vi "读取数据文件-扭转.vi"(0 "文件路径（使用对话框）":path) -> (1 "第一列":dbl[](array[numeric]), 2 "第二列":dbl[](array[numeric]))   [LabVIEW 2016]
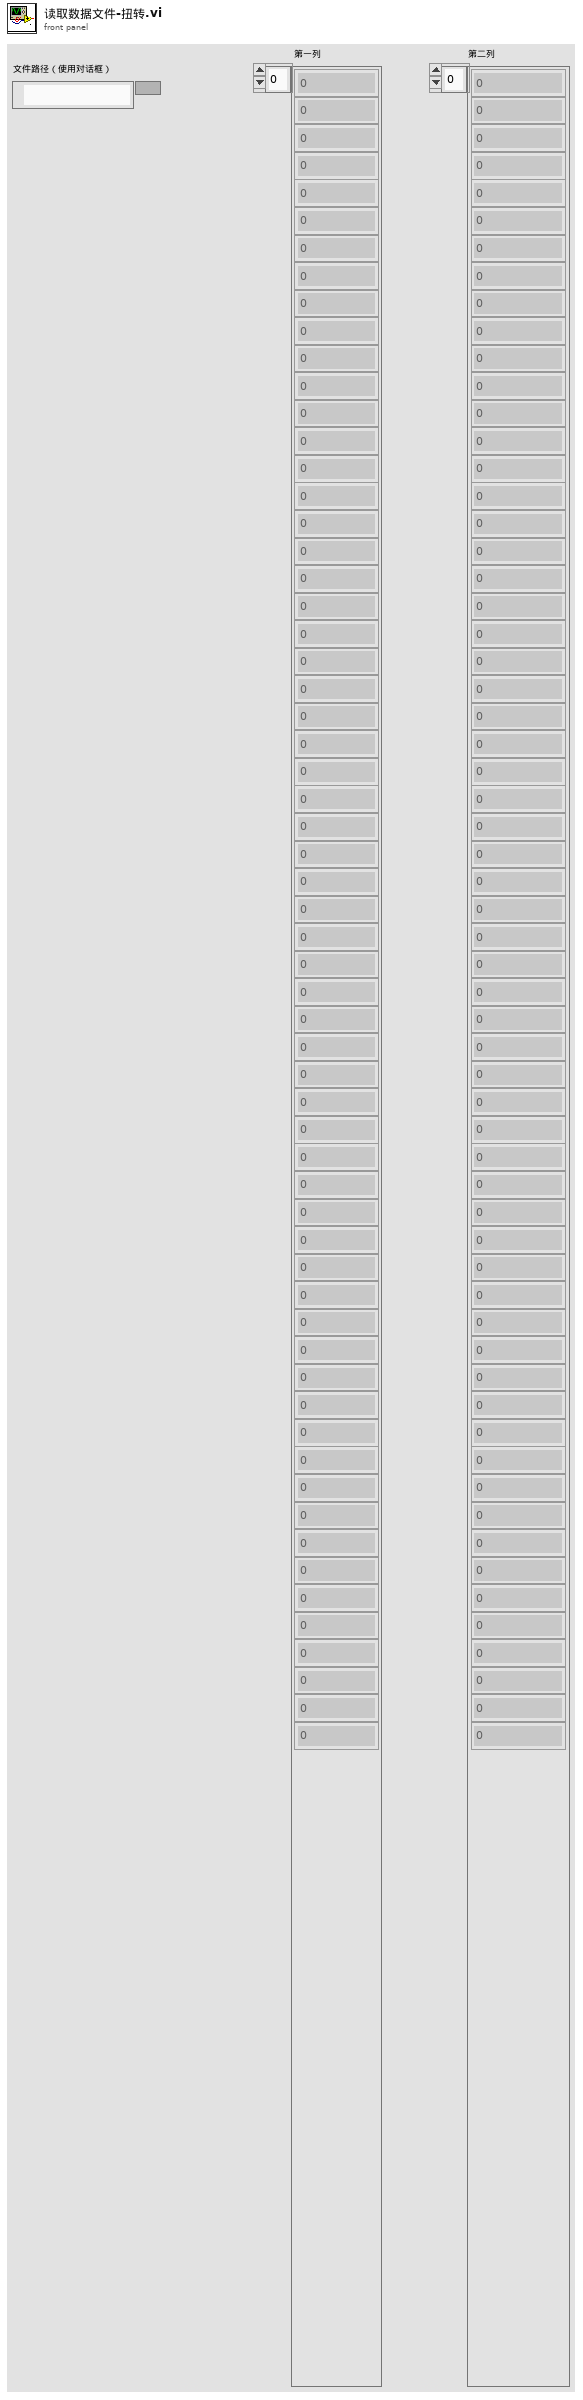
[diagram p1: front panel]
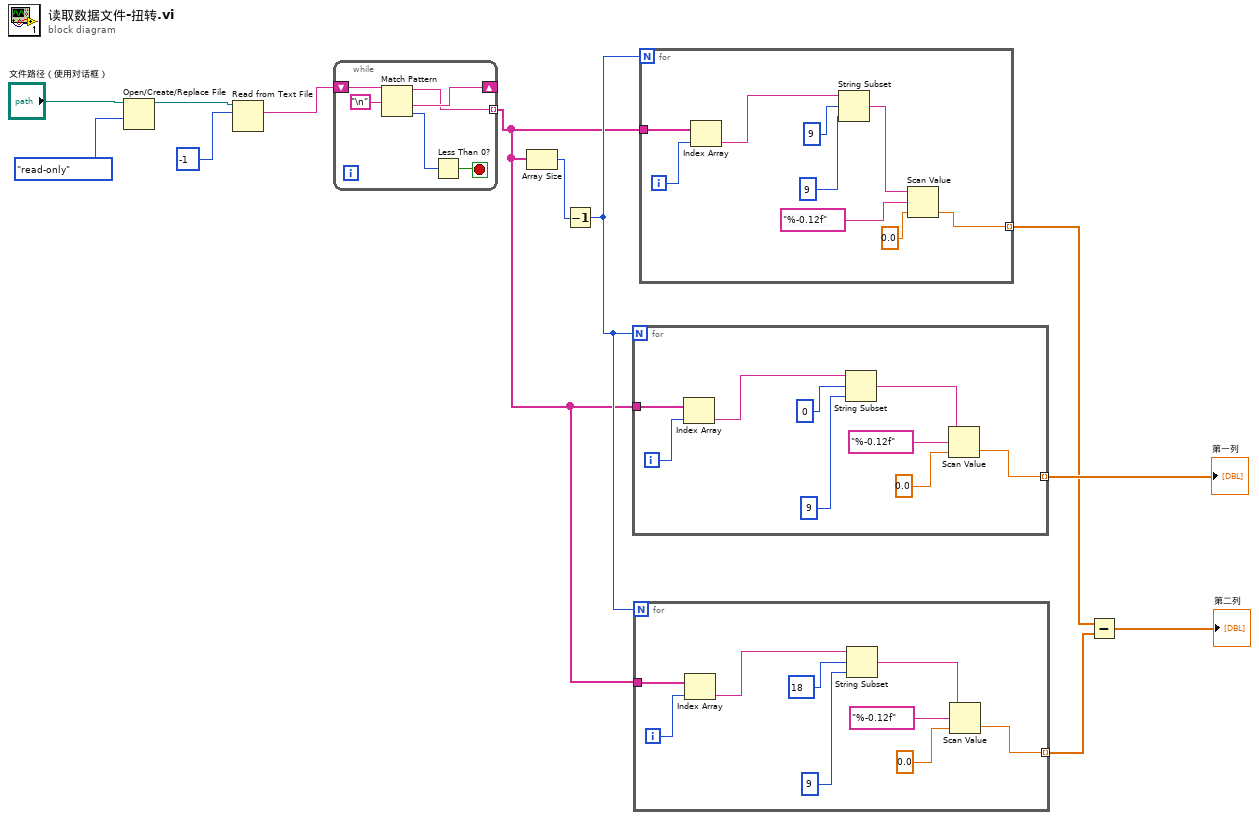
[diagram p0: block diagram]
diagram:
  n1 = Open/Create/Replace File(file path (use dialog)="文件路径（使用对话框）", access (0:read/write)=enum16{"read/write", "read-only", "write-only"}."read-only" ("权限(0:read/write)")) -> (refnum out=w10:refnum<file>)  [unwired: 4 in, 2 out]
  n2 = Read from Text File(file (use dialog)=w10, count=-1 ("计数")) -> (text=w8:string)  [unwired: 2 in, 3 out]
  n3 = while {
    tunnel: [w13] -> w4 mode=indexing
    shift-right: [w16] -> _
    shift-left: w8 -> [w17]
    stop <- w15 stop-if-true
    n4 = Match Pattern(string=w17, regular expression="\n") -> (before substring=w13:string, after substring=w16:string, offset past match=w14:i32)  [unwired: 1 in, 1 out]
    n5 = Less Than 0?(x=w14) -> (x < 0?=w15:bool)
  }
  n6 = Array Size(array=w4) -> (size(s)=w7:i32)
  n7 = Decrement(x=w7) -> (x-1=w5:i32)
  n8 = for {
    N: w5 -> [_]
    tunnel: w4 -> [w27]
    tunnel: [w19] -> w6 mode=indexing
    i -> [w26]
    n9 = Index Array(array=w27, index=w26) -> (element=w25:string)
    n10 = String Subset(string=w25, offset (0)=0 ("偏移量(0)"), length (rest)=9 ("长度（剩余）")) -> (substring=w20:string)
    n11 = Scan Value(string=w20, format string="%-0.12f" ("格式字符串"), default (0 dbl)=0.0 ("默认(0 dbl)")) -> (value=w19:dbl)  [unwired: 1 out]
  }
  "第一列" <- w6
  n12 = for {
    N: w5 -> [_]
    tunnel: w4 -> [w36]
    tunnel: [w28] -> w2 mode=indexing
    i -> [w35]
    n13 = Index Array(array=w36, index=w35) -> (element=w34:string)
    n14 = String Subset(string=w34, offset (0)=18 ("偏移量(0)"), length (rest)=9 ("长度（剩余）")) -> (substring=w29:string)
    n15 = Scan Value(string=w29, format string="%-0.12f" ("格式字符串"), default (0 dbl)=0.0 ("默认(0 dbl)")) -> (value=w28:dbl)  [unwired: 1 out]
  }
  n16 = for {
    N: w5 -> [_]
    tunnel: w4 -> [w45]
    tunnel: [w37] -> w3 mode=indexing
    i -> [w44]
    n17 = Index Array(array=w45, index=w44) -> (element=w43:string)
    n18 = String Subset(string=w43, offset (0)=9 ("偏移量(0)"), length (rest)=9 ("长度（剩余）")) -> (substring=w40:string)
    n19 = Scan Value(string=w40, format string="%-0.12f" ("格式字符串"), default (0 dbl)=0.0 ("默认(0 dbl)")) -> (value=w37:dbl)  [unwired: 1 out]
  }
  n20 = Subtract(x=w3, y=w2) -> (x-y=→"第二列":dbl[])
